vi "ShowBar.vi"(0 "This VI":refnum<vi>) -> ()   [LabVIEW 2018]
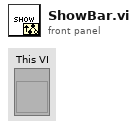
[diagram p1: front panel]
types:
  T1 = enum32{"invalid app kind", "Development System", "Run Time System", "Student Edition", "Embedded LabVIEW", "Evaluation", "Custom"}
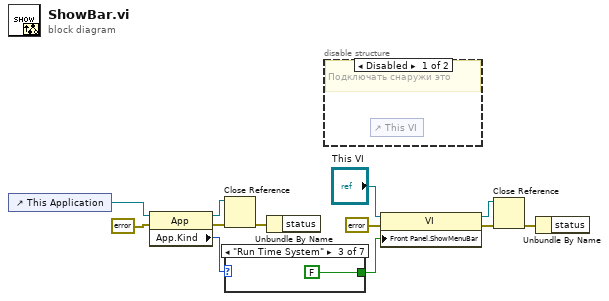
[diagram p0: block diagram]
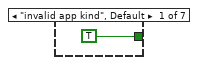
[diagram p3: hidden frame]
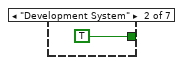
[diagram p4: hidden frame]
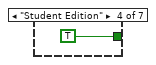
[diagram p5: hidden frame]
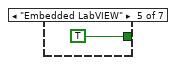
[diagram p6: hidden frame]
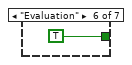
[diagram p7: hidden frame]
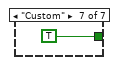
[diagram p8: hidden frame]
diagram:
  n1 = control-ref of="This Application"() -> (w1:refnum<vi>)
  n2 = property class="App"(reference=w1, error in=errorcluster {"status"=FALSE, "code"=0, "source"=""} ("error in (no error)")) -> (reference out=w2:refnum<vi>, error out=w3:errorcluster, "App.Kind"=w12:T1)
  n3 = Close Reference(reference=w2, error in (no error)=w3) -> (error out=w4:errorcluster)
  n4 = case shown="\"Run Time System\"" w12 {
    tunnel: [TRUE TRUE FALSE TRUE TRUE TRUE TRUE] -> w11
    frame "invalid app kind", Default {
    }
    frame "Development System" {
    }
    frame "Run Time System" {
    }
    frame "Student Edition" {
    }
    frame "Embedded LabVIEW" {
    }
    frame "Evaluation" {
    }
    frame "Custom" {
    }
  }
  n5 = Unbundle By Name(w4) -> ()  [unwired: 1 out]
  n6 = disable-structure shown="Disabled" {
    frame Disabled {
      # "Подключать снаружи это"
      n7 = control-ref of="This VI"() -> ()  [unwired: 1 out]
    }
    frame Enabled {
    }
  }
  n8 = property class="VI"(reference="This VI", error in=errorcluster {"status"=FALSE, "code"=0, "source"=""} ("error in (no error)"), "Front Panel.ShowMenuBar"=w11) -> (reference out=w6:refnum<vi>, error out=w7:errorcluster)
  n9 = Close Reference(reference=w6, error in (no error)=w7) -> (error out=w5:errorcluster)
  n10 = Unbundle By Name(w5) -> ()  [unwired: 1 out]
